vi "Lean Angle Measurement.vi"(9 "Lean angle offset":dbl=2.2 format="%#_13g", 11 "error in (no error)":errorcluster) -> (2 "Output":T1, 3 "error out":errorcluster)   [LabVIEW 2016]
uses:
  <vilib>/myRIO/Instrument Drivers/Onboard IO/UART/typedef/VISA Configuration.ctl
  <vilib>/Instr/_visa.llb/VISA Configure Serial Port (Instr).vi
  <vilib>/myRIO/Express VI/Onboard IO/UART/UART Express VI.xnode
  <vilib>/myRIO/Instrument Drivers/Onboard IO/UART/UART.lvlib
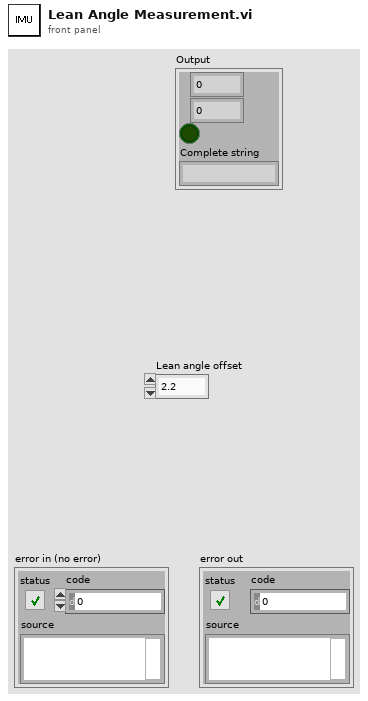
[diagram p1: front panel]
types:
  T1 = cluster{dbl, dbl, bool, "Complete string":string}
  T2 = cluster{dbl, dbl, bool, "Characters Read":string}
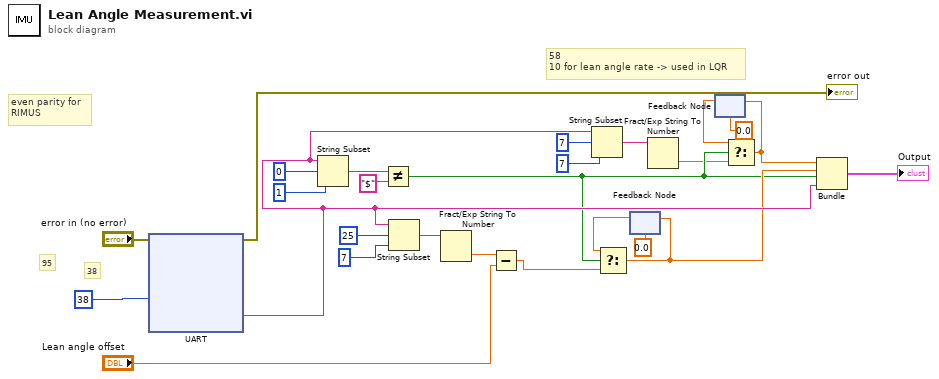
[diagram p0: block diagram]
diagram:
  # "58\n10 for lean angle rate -> used in LQR"
  # "even parity for \nRIMUS"
  # "38"
  # "95"
  n1 = xnode "UART"("Character Count"=u32 38, "error in (no error)"="error in (no error)") -> ("Characters Read"=w13:string, "error out"=→"error out":errorcluster)
  n2 = String Subset(string=w13, offset (0)=0 ("length (rest)"), length (rest)=1 ("length (rest)")) -> (substring=w22:string)
  n3 = Not Equal?(x=w22, y="$") -> (x != y?=w5:bool)
  n4 = String Subset(string=w13, offset (0)=25, length (rest)=7 ("length (rest)")) -> (substring=w24:string)
  n5 = Fract/Exp String To Number(string=w24) -> (number=w17:dbl)  [unwired: 3 in, 1 out]
  n6 = Subtract(x=w17, y="Lean angle offset") -> (x-y=w9:dbl)
  n7 = String Subset(string=w13, offset (0)=7, length (rest)=7 ("length (rest)")) -> (substring=w14:string)
  n8 = feedback #1(0.0) -> (w7:dbl)
  n9 = Select(t=w7, s=w5, f=w9) -> (s? t:f=w8:dbl)
  n10 = feedback-in #1(w8) -> ()
  n11 = Fract/Exp String To Number(string=w14) -> (number=w4:dbl)  [unwired: 3 in, 1 out]
  n12 = feedback #2(0.0) -> (w2:dbl)
  n13 = Select(t=w2, s=w5, f=w4) -> (s? t:f=w3:dbl)
  n14 = feedback-in #2(w3) -> ()
  n15 = Bundle(w3, w8, w5, "Characters Read"=w13) -> (→"Output":T2)  [unwired: 1 in]
